vi "Table Mouse Move.vi"(5 "On Color":u32(colorbox)=10551291, 7 "Off Color":u32(colorbox)=16448250, 8 "error in":errorcluster, 9 "Previous Cell Position":T2={"Row"=-2, "Column"=-2}, 10 "Coords In":T1, 11 "Table Ref In":refnum<vi>) -> (0 "error out":errorcluster, 1 "Cell Position":T2, 3 "Table Ref Out":refnum<vi>)   [LabVIEW 2024]
uses:
  <vilib>/Utility/miscctls.llb/LVRowAndColumnTypeDef.ctl
  <vilib>/Utility/miscctls.llb/LVPoint32TypeDef.ctl
  <vilib>/Utility/miscctls.llb/LVPositionTypeDef.ctl
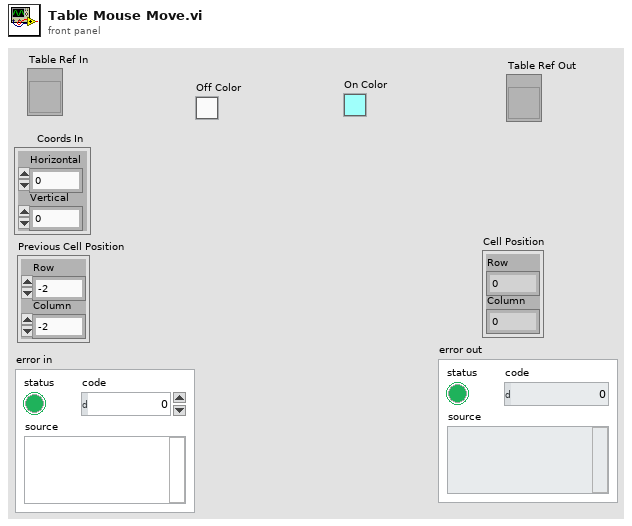
[diagram p1: front panel]
types:
  T1 = typedef "LVPoint32TypeDef.ctl" = cluster{"Horizontal":i32, "Vertical":i32}
  T2 = typedef "LVRowAndColumnTypeDef.ctl" = cluster{"Row":i32, "Column":i32}
  T3 = typedef "LVPositionTypeDef.ctl" = cluster{"Left":i32, "Top":i32}
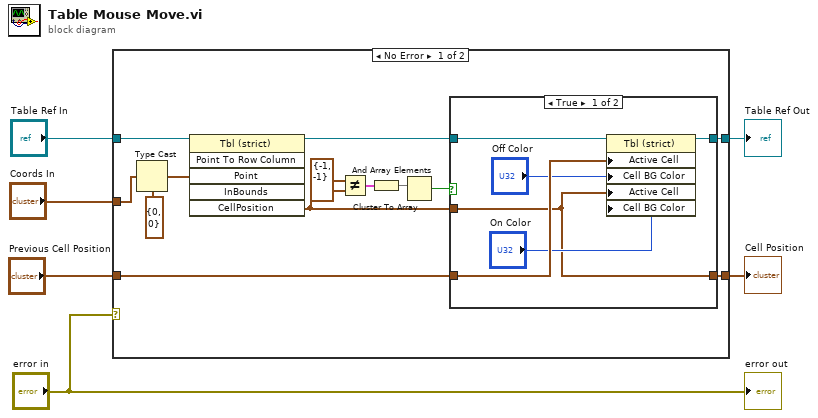
[diagram p0: block diagram]
diagram:
  n1 = case shown="No Error" "error in" {
    tunnel: "Table Ref In" -> [w11 w29]
    tunnel: [w10 w29] -> w5
    tunnel: "Previous Cell Position" -> [w9 w28]
    tunnel: [w8 w28] -> w3
    tunnel: "Coords In" -> [w7 _]
    frame No Error {
      n2 = Type Cast(type=T3 {"Left"=0, "Top"=0} ("Point"), x=w7) -> (*(type *) &x=w18:T3)
      n3 = invoke class="Tbl (strict)" method="Point To Row Column"(reference=w11, "Point"=w18) -> (reference out=w17:refnum<vi>, "CellPosition"=w16:T2)  [unwired: 4 in, 4 out]
      n4 = Not Equal?(x=T2 {"Row"=-1, "Column"=-1}, y=w16) -> (x != y?=w14:cluster{"Row":bool, "Column":bool})
      n5 = Cluster To Array(cluster=w14) -> (array=w12:bool[])
      n6 = And Array Elements(Boolean array=w12) -> (logical AND=w13:bool)
      n7 = case shown="True" w13 {
        tunnel: w17 -> [w25 w26]
        tunnel: w9 -> [w24 w27]
        tunnel: w16 -> [w21 _]
        tunnel: [w21 w27] -> w8
        tunnel: [w20 w26] -> w10
        frame True {
          n8 = property class="Tbl (strict)"(reference=w25, "Active Cell"=w24, "Cell BG Color"="Off Color", "Active Cell"=w21, "Cell BG Color"="On Color") -> (reference out=w20:refnum<vi>)  [unwired: 1 in, 1 out]
        }
        frame False {
        }
      }
    }
    frame Error {
    }
  }
  "Table Ref Out" <- w5
  "Cell Position" <- w3
  "error out" <- "error in"
